vi "user output.vi"(8 "error in":errorcluster, 11 "Outputs to system":T1) -> (0 "error out":errorcluster)   [LabVIEW 2017, in "ScaleAndLimitModule runtime.lvclass"]
uses:
  ScaleAndLimitModule runtime.lvclass
  output user data.ctl
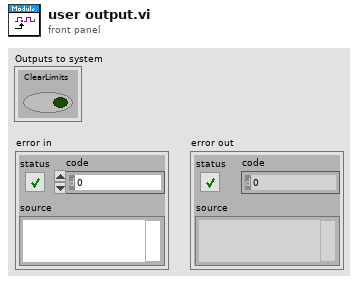
[diagram p1: front panel]
types:
  T1 = typedef "ScaleAndLimitModule runtime.lvclass/output user data.ctl" = cluster{"ClearLimits":bool}
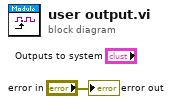
[diagram p0: block diagram]
diagram:
  "error out" <- "error in"
